vi "colorir_campo.vi"(8 "ID":i32, 9 "grid y":i32=181, 10 "grid x":i32=121, 11 "3D Probability Matrix":dbl[][][](array[numeric])) -> (1 "campo colorido":picture)   [LabVIEW 2017]
uses:
  <vilib>/picture/picture.llb/Draw True-Color Pixmap.vi
  <vilib>/Utility/file.llb/Read Delimited Spreadsheet (string).vi
panel:
  out "all rows":string[][](array[string])
  in  "file path (dialog if empty)":path
  in  "path to PNG file":path=path "C:/Users/Robótica/git/SSL-SOS/SOS/field.png"
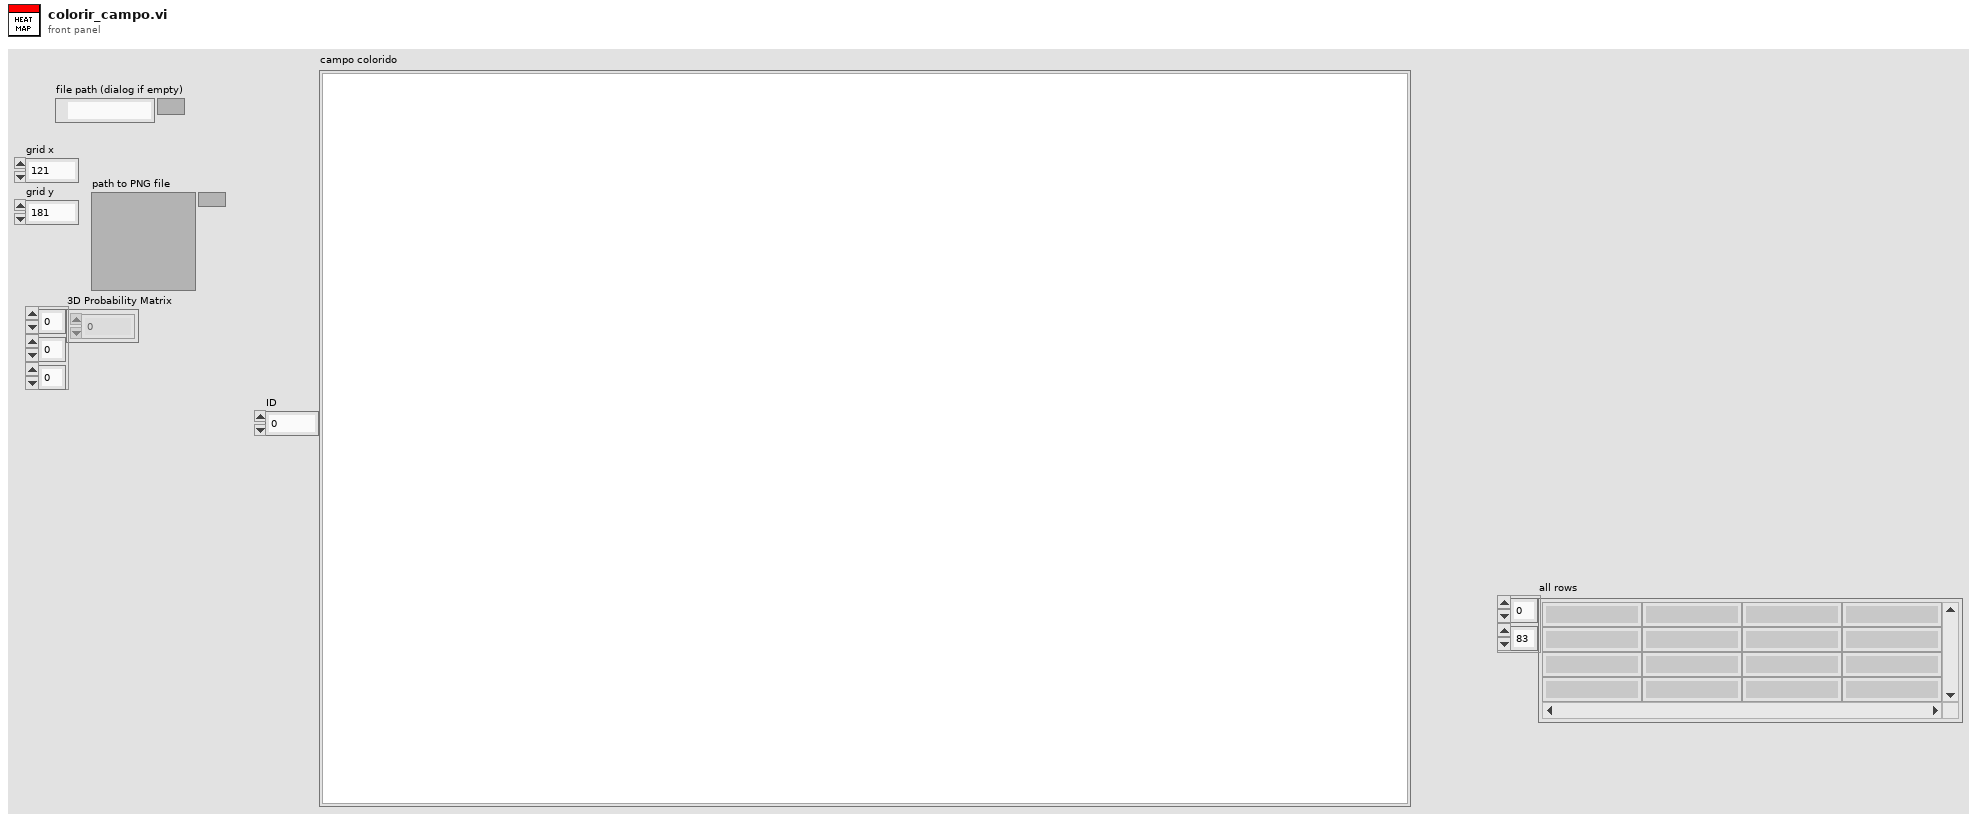
[diagram p1: front panel]
types:
  T1 = typedef "imagedata.ctl" = cluster{"image type":i32, "image depth":i32, "image":u8[], "mask":u8[], "colors":u32[], "Rectangle":cluster{"left":i16, "top":i16, "right":i16, "bottom":i16}}
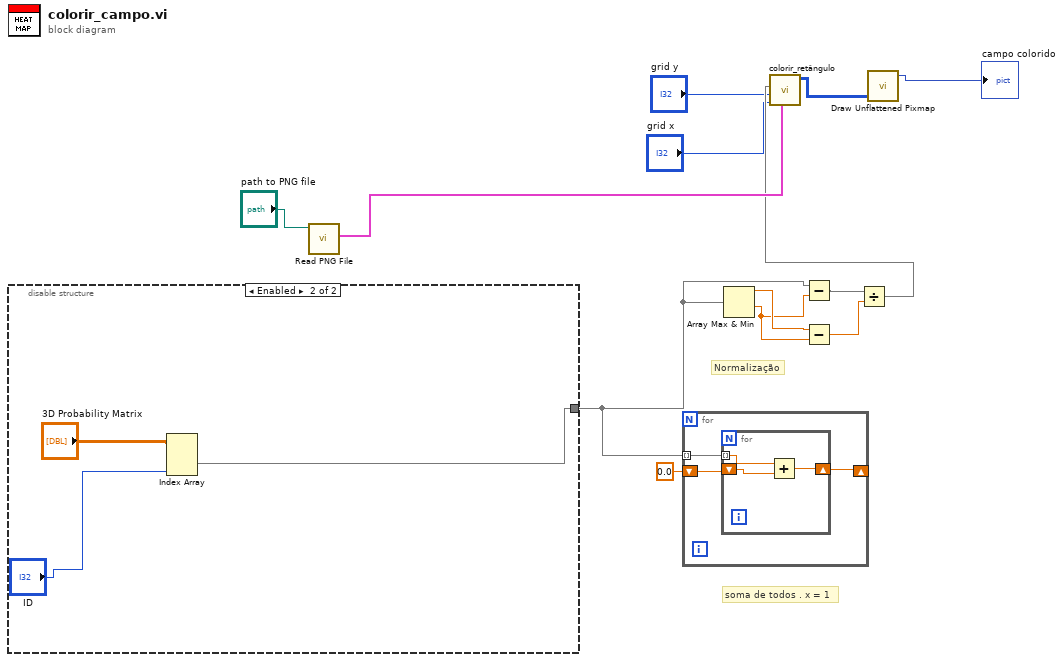
[diagram p0: block diagram]
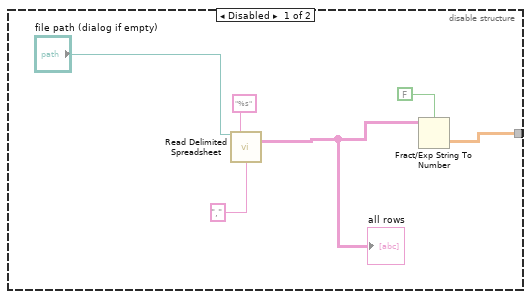
[diagram p2: hidden frame]
diagram:
  # "soma de todos . x = 1"
  # "Normalização"
  n1 = disable-structure shown="Enabled" {
    disable-tunnel: [w14 w21] -> w3
    frame Disabled {
      n2 = call-poly <vilib>:"Read Delimited Spreadsheet.vi"("file path (dialog if empty)"="file path (dialog if empty)", "format (%s)"="%s" ("format (%.3f)"), "delimiter (\\t)"="," ("delimiter (\\t)")) -> ("all rows"=w16:string[][])  [unwired: 7 in, 5 out]
      "all rows" <- w16
      n3 = Fract/Exp String To Number(use system decimal point (T)=FALSE, string=w16) -> (number=w14:dbl[][])  [unwired: 2 in, 1 out]
    }
    frame Enabled {
      n4 = Index Array(array="3D Probability Matrix", index (dim 2)="ID") -> (element=w21:dbl[][])  [unwired: 2 in]
    }
  }
  n5 = call <vilib>:"Read PNG File.vi"("path to PNG file"="path to PNG file") -> ("image data"=w12:T1)  [unwired: 8 in, 2 out]
  n6 = for {
    tunnel: w3 -> [w25] mode=indexing
    shift-right: [w24] -> _
    shift-left: 0.0 -> [w23]
    n7 = for {
      tunnel: w25 -> [w28] mode=indexing
      shift-right: [w27] -> w24
      shift-left: w23 -> [w26]
      n8 = Add(x=w28, y=w26) -> (x+y=w27:dbl)
    }
  }
  n9 = Array Max & Min(array=w3) -> (max value=w9:dbl, min value=w8:dbl)  [unwired: 2 out]
  n10 = Subtract(x=w3, y=w8) -> (x-y=w2:dbl[][])
  n11 = Subtract(x=w9, y=w8) -> (x-y=w1:dbl)
  n12 = Divide(x=w2, y=w1) -> (x/y=w7:dbl[][])
  n13 = call "colorir_retângulo.vi"("image data"=w12, "m (colunas)"="grid x", "n (linhas)"="grid y", "Matriz de probabilidades"=w7) -> ("data out"=w11:u32[][])  [unwired: 7 in]
  n14 = call-poly <vilib>:"Draw Unflattened Pixmap.vi"("data (RGB format)"=w11) -> ("new picture"=→"campo colorido":picture)  [unwired: 8 in]
